vi "Create Hue Array.vi"(8 "error in (no error)":errorcluster, 11 "ColorSelector in":refnum<class "ColorSelector.lvclass">) -> (0 "error out":errorcluster, 3 "ColorSelector out":refnum<class "ColorSelector.lvclass">)   [LabVIEW 2015, in "ColorSelector.lvclass"]
doc: "This VI creates the initial Hue array.\n<b> </b> <b> </b>\n©2017 Q Software Innovations, LLC (QSI)\nwritten by Quentin Alldredge\nproduced in LabVIEW 2015\n\nsupport@qsoftwareinnovations.com\nwww.qsoftwareinnovations.com\n\nAll rights reserved.\n\nRedistribution and use in source and binary forms, with or without modification, are permitted provided that the following conditions are met:\n\n * Redistributions of source code must retain the above copyright notice, this list of conditions and the following disclaimer.\n * Redistributions in binary form must reproduce the above copyright notice, this list of conditions and the following disclaimer in the documentation and/or other materials provided with the distribution.\n * Neither the name of Q Software Innovations, LLC. nor the names of its contributors may be used to endorse or promote products derived from this software without specific prior written permission.\n\nTHIS SOFTWARE IS PROVIDED BY THE COPYRIGHT HOLDERS AND CONTRIBUTORS \"AS IS\" AND ANY EXPRESS OR IMPLIED WARRANTIES, INCLUDING, BUT NOT LIMITED TO, THE IMPLIED WARRANTIES OF MERCHANTABILITY AND FITNESS FOR A PARTICULAR PURPOSE ARE DISCLAIMED. IN NO EVENT SHALL THE COPYRIGHT OWNER OR CONTRIBUTORS BE LIABLE FOR ANY DIRECT, INDIRECT, INCIDENTAL, SPECIAL, EXEMPLARY, OR CONSEQUENTIAL DAMAGES (INCLUDING, BUT NOT LIMITED TO, PROCUREMENT OF SUBSTITUTE GOODS OR SERVICES; LOSS OF USE, DATA, OR PROFITS; OR BUSINESS INTERRUPTION) HOWEVER CAUSED AND ON ANY THEORY OF LIABILITY, WHETHER IN CONTRACT, STRICT LIABILITY, OR TORT (INCLUDING NEGLIGENCE OR OTHERWISE) ARISING IN ANY WAY OUT OF THE USE OF THIS SOFTWARE, EVEN IF ADVISED OF THE POSSIBILITY OF SUCH DAMAGE."
uses:
  ColorSelector.lvclass
  ColorSelector.lvclass/ColorSelector.ctl
  Write Hue[].vi
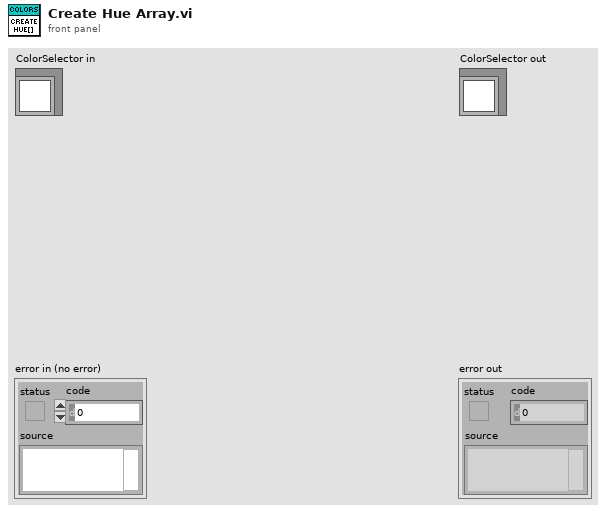
[diagram p1: front panel]
types:
  T1 = typedef "LVBoundsTypeDef.ctl" = cluster{"Width":u32, "Height":u32}
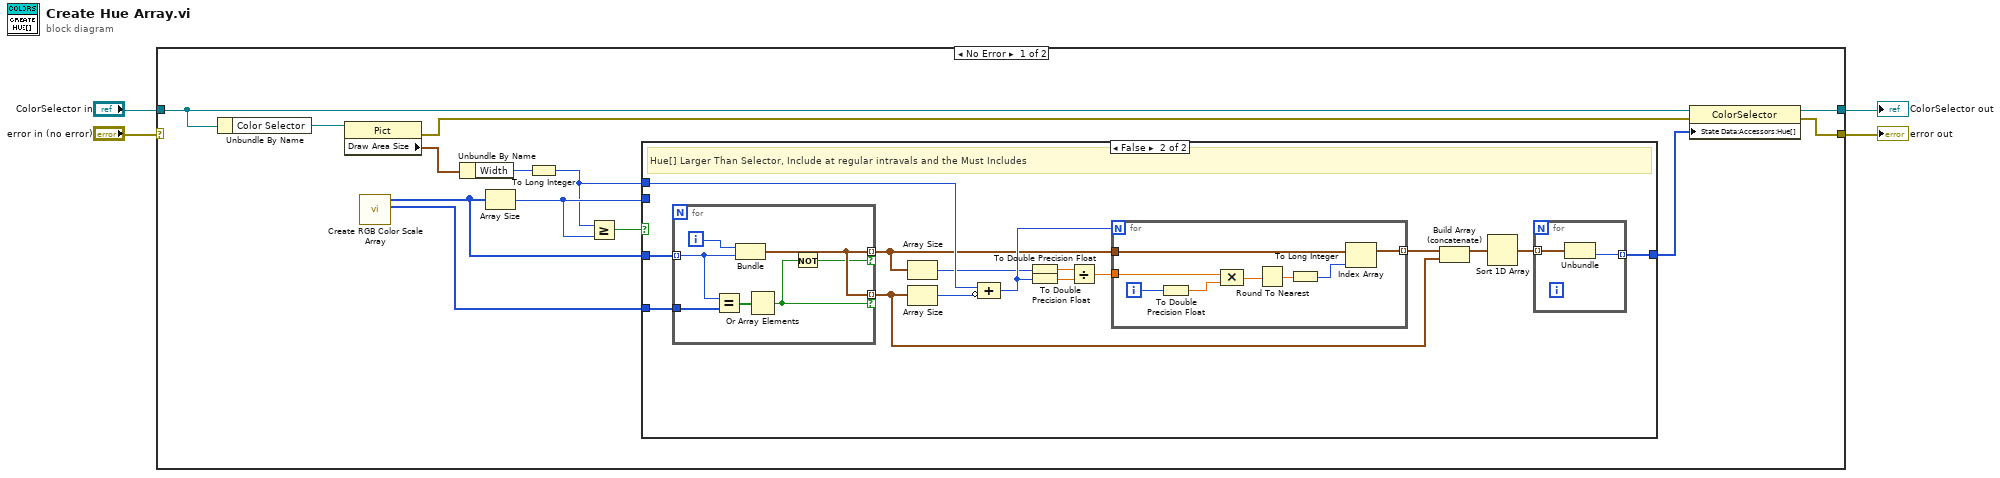
[diagram p0: block diagram]
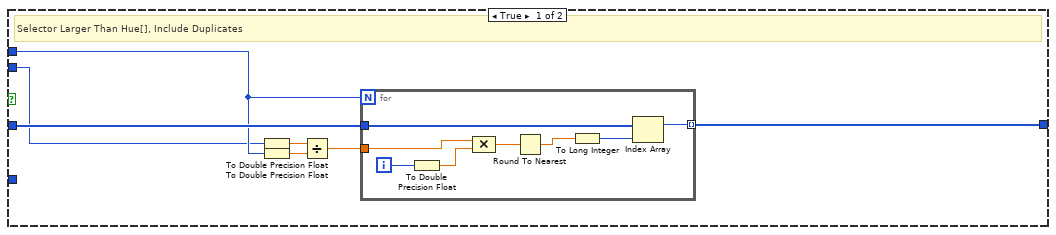
[diagram p2: hidden frame]
diagram:
  n1 = case shown="No Error" "error in (no error)" {
    selector: "error in (no error)" -> [_ w66]
    tunnel: [w8 w66] -> w3
    tunnel: [w11 w65] -> w1
    tunnel: "ColorSelector in" -> [w12 w65]
    frame No Error {
      n2 = Unbundle By Name(w12) -> ("Color Selector"=w17:refnum<vi>)
      n3 = property on="Property Node" class="Pict"(reference=w17) -> (error out=w10:errorcluster, "Draw Area Size"=w13:T1)  [unwired: 1 in, 1 out]
      n4 = call "Create RGB Color Scale Array.vi"() -> ("RGB Must Include"=w5:u32[], "RGB Array"=w6:u32[])  [unwired: 10 in]
      n5 = Unbundle By Name(w13) -> ("Width"=w14:u32)
      n6 = Array Size(array=w6) -> (size(s)=w16:i32)
      n7 = To Long Integer(number=w14) -> (32bit integer=w7:i32)
      n8 = Greater Or Equal?(x=w7, y=w16) -> (x >= y?=w15:bool)
      n9 = case shown="False" w15 {
        tunnel: w6 -> [w20 w41]
        tunnel: [w24 w42] -> w9
        tunnel: w7 -> [w19 w39]
        tunnel: w16 -> [w18 _]
        tunnel: w5 -> [_ w33]
        frame True {
          # "Selector Larger Than Hue[], Include Duplicates"
          n10 = To Double Precision Float(number=w18) -> (double precision float=w22:dbl)
          n11 = To Double Precision Float(number=w19) -> (double precision float=w21:dbl)
          n12 = Divide(x=w22, y=w21) -> (x/y=w23:dbl)
          n13 = for {
            N: w19 -> [_]
            tunnel: w20 -> [w32]
            tunnel: [w27] -> w24 mode=indexing
            tunnel: w23 -> [w31]
            i -> [w28]
            n14 = To Double Precision Float(number=w28) -> (double precision float=w26:dbl)
            n15 = Compound Arithmetic op=MULTIPLY(w31, w26) -> (w30:dbl)
            n16 = Round To Nearest(number=w30) -> (nearest integer value=w29:dbl)
            n17 = To Long Integer(number=w29) -> (32bit integer=w25:i32)
            n18 = Index Array(array=w32, index=w25) -> (element=w27:u32)
          }
        }
        frame False {
          # "Hue[] Larger Than Selector, Include at regular intravals and the Must Includes"
          n19 = for {
            tunnel: w41 -> [w51] mode=indexing
            tunnel: [w53] -> w35 mode=indexing if=w48
            tunnel: [w53] -> w38 mode=indexing if=w49
            tunnel: w33 -> [w52]
            i -> [w54]
            n20 = Equal?(x=w51, y=w52) -> (x = y?=w50:bool[])
            n21 = Bundle(w54, "Color"=w51) -> (w53:cluster{i32, "Color":u32})  [unwired: 1 in]
            n22 = Or Array Elements(Boolean array=w50) -> (logical OR=w49:bool)
            n23 = Not(x=w49) -> (.not. x?=w48:bool)
          }
          n24 = Array Size(array=w35) -> (size(s)=w34:i32)
          n25 = Array Size(array=w38) -> (size(s)=w37:i32)
          n26 = Compound Arithmetic op=ADD(w39, invert w37) -> (w36:i32)
          n27 = To Double Precision Float(number=w34) -> (double precision float=w45:dbl)
          n28 = To Double Precision Float(number=w36) -> (double precision float=w44:dbl)
          n29 = Divide(x=w45, y=w44) -> (x/y=w46:dbl)
          n30 = for {
            N: w36 -> [_]
            tunnel: w35 -> [w59]
            tunnel: [w57] -> w47 mode=indexing
            tunnel: w46 -> [w64]
            i -> [w63]
            n31 = To Double Precision Float(number=w63) -> (double precision float=w62:dbl)
            n32 = Compound Arithmetic op=MULTIPLY(w64, w62) -> (w60:dbl)
            n33 = Round To Nearest(number=w60) -> (nearest integer value=w61:dbl)
            n34 = To Long Integer(number=w61) -> (32bit integer=w58:i32)
            n35 = Index Array(array=w59, index=w58) -> (element=w57:cluster{i32, "Color":u32})
          }
          n36 = Build Array (concatenate)(w47, w38) -> (w43:cluster{i32, "Color":u32}[])
          n37 = Sort 1D Array(array=w43) -> (sorted array=w40:cluster{i32, "Color":u32}[])
          n38 = for {
            tunnel: w40 -> [w56] mode=indexing
            tunnel: [w55] -> w42 mode=indexing
            n39 = Unbundle(w56) -> ("Color"=w55:u32)  [unwired: 1 out]
          }
        }
      }
      n40 = property class="ColorSelector"(reference=w12, error in=w10, "State Data:Accessors:Hue[]"=w9) -> (reference out=w11:refnum<class "ColorSelector.lvclass">, error out=w8:errorcluster)
    }
    frame Error {
    }
  }
  "error out" <- w3
  "ColorSelector out" <- w1
